vi "AW_Calculate_Tester_Parameter_Initialisation.vi"(9 "Tester Parameter":dbl[](array[numeric]), 11 "DDM Parameter":dbl[](array[numeric])) -> (3 "Calculate Tester Parameter":dbl[](array[numeric]))   [LabVIEW 2017]
panel:
  out "delta_v":dbl
  out "ddm_real_power":dbl
  out "DDM Pressure":dbl
  out "DDM Speed":dbl
  out "DDM Power":dbl
  out "DDM Current":dbl
  out "DDM Voltage":dbl
  out "Ambient humidity":dbl
  out "Ambient temperature":dbl
  out "Ambient pressure":dbl
  out "power":dbl
  out "current":dbl
  out "voltage":dbl
  out "DDM_Pressure_corrected":dbl
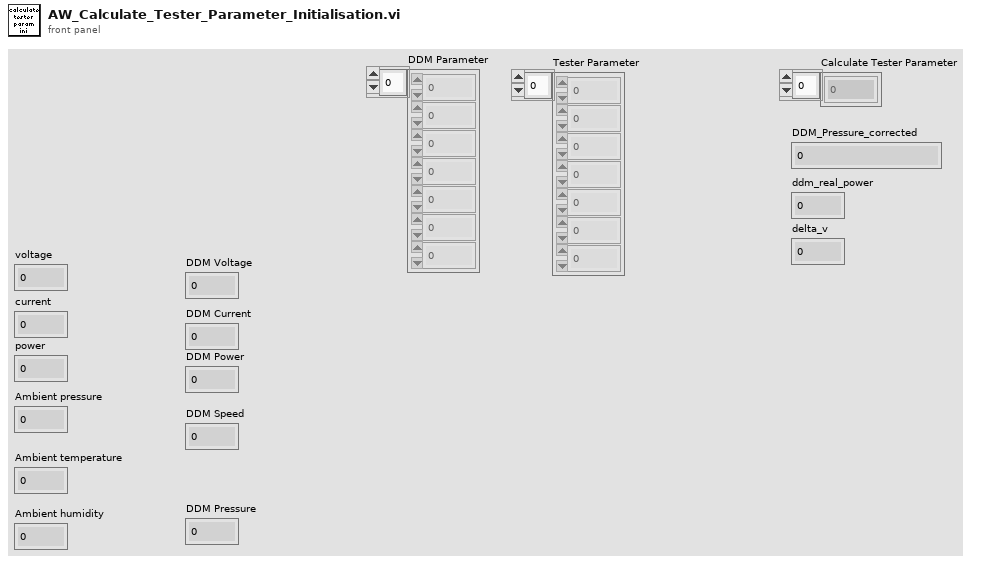
[diagram p1: front panel]
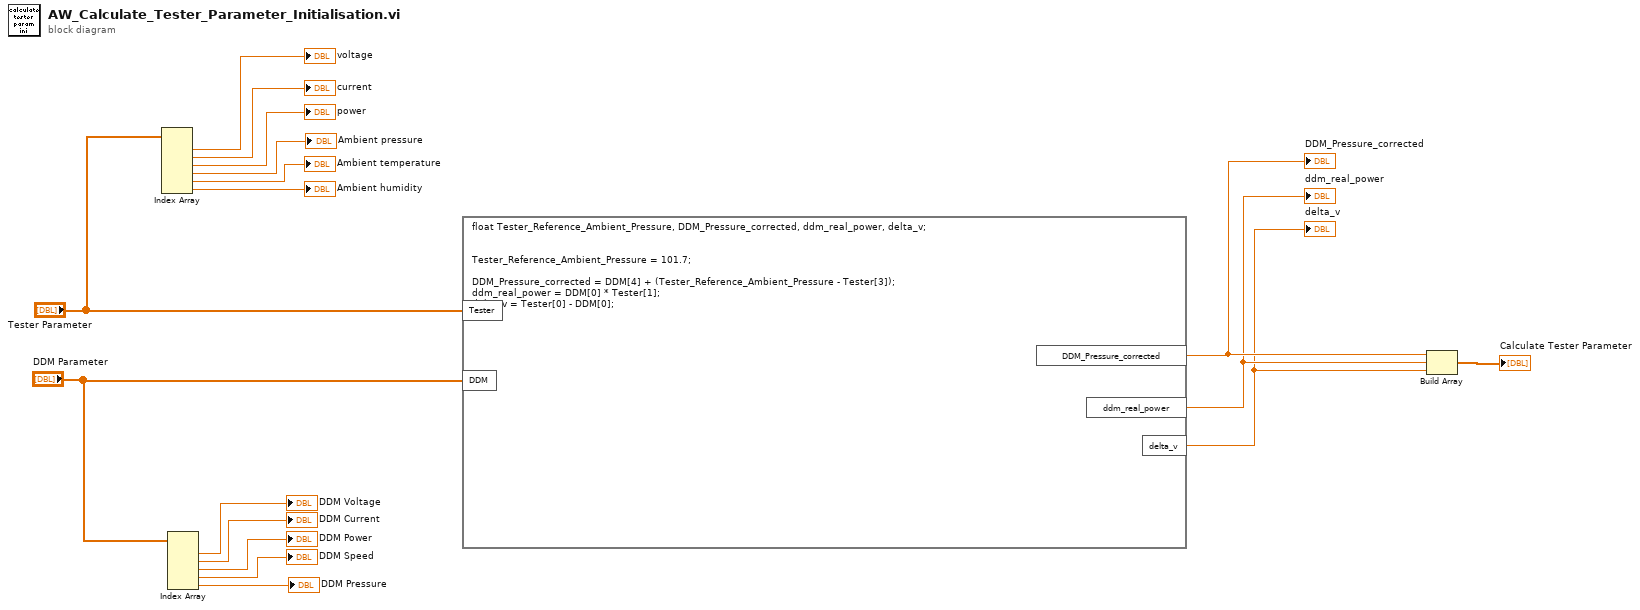
[diagram p0: block diagram]
diagram:
  n1 = Index Array(array="Tester Parameter") -> (element #1=→"voltage":dbl, element #2=→"current":dbl, element #3=→"power":dbl, element #4=→"Ambient pressure":dbl, element #5=→"Ambient temperature":dbl, element #6=→"Ambient humidity":dbl)  [unwired: 6 in]
  n2 = Index Array(array="DDM Parameter") -> (element #1=→"DDM Voltage":dbl, element #2=→"DDM Current":dbl, element #3=→"DDM Power":dbl, element #4=→"DDM Speed":dbl, element #5=→"DDM Pressure":dbl)  [unwired: 5 in]
  n3 = formula code="float Tester_Reference_Ambient_Pressure, DDM_Pressure_corrected, ddm_real_power, delta_v;\n\n\nTester_Reference_Ambient_Pressure = 101.7;\n\nDDM_Pressure_corrected = DDM[4] + (Tester_Reference_Ambient_Pressure - Tester[3]);\nddm_real_power = DDM[0] * Tester[1];\ndelta_v = Tester[0] - DDM[0];"("Tester"="Tester Parameter", "DDM"="DDM Parameter") -> ("DDM_Pressure_corrected"=w5:dbl, "ddm_real_power"=w4:dbl, "delta_v"=w3:dbl)
  "DDM_Pressure_corrected" <- w5
  "ddm_real_power" <- w4
  "delta_v" <- w3
  n4 = Build Array(w5, w4, w3) -> (→"Calculate Tester Parameter":dbl[])
